vi "CUDA Toolkit Not Complex Graph.vi"(7 "nb_loop":i32=5, 8 "error in (no error)":errorcluster, 10 "B":refnum<class "Tensor.lvclass">, 11 "A":refnum<class "Tensor.lvclass">) -> (0 "error out":errorcluster, 3 "sum":sgl)   [LabVIEW 2020]
uses:
  Cuda/Source/Tensor.lvclass
  Cuda/Source/Methods/Functions/Numeric/SGL/Add Array Scalar(SGL).vi
  Cuda/Source/Methods/Functions/Numeric/SGL/Multiply Array Array(SGL).vi
  Cuda/Source/Methods/Functions/Numeric/SGL/Divide Array Array(SGL).vi
  Cuda/Source/Methods/Functions/Numeric/SGL/Add Array Element(SGL).vi
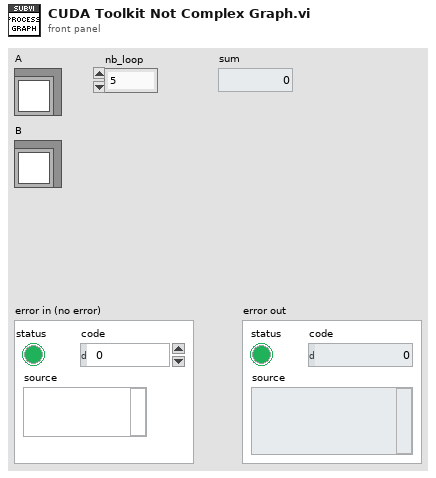
[diagram p1: front panel]
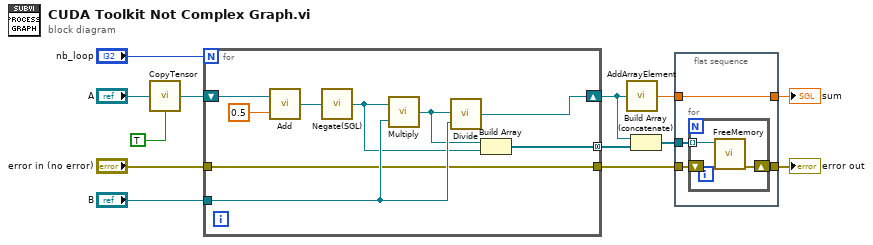
[diagram p0: block diagram]
diagram:
  n1 = call "CopyTensor.vi"("Tensor Src"="A", "copy data ?"=TRUE) -> ("Tensor Dst"=w9:refnum<class "Tensor.lvclass">)  [unwired: 13 in]
  n2 = for {
    N: "nb_loop" -> [_]
    tunnel: "B" -> [w20]
    shift-right: [w19] -> w5
    shift-left: w9 -> [w21]
    tunnel: "error in (no error)" -> [w17]
    tunnel: [w17] -> w7
    tunnel: [w14] -> w4 mode=concatenating
    n3 = call-poly "Add.vi"("y"=sgl 0.5, "x"=w21) -> ("x + y"=w18:refnum<class "Tensor.lvclass">)
    n4 = call "Negate(SGL).vi"("x"=w18) -> ("-x"=w15:refnum<class "Tensor.lvclass">)
    n5 = call-poly "Multiply.vi"("y"=w20, "x"=w15) -> ("x * y"=w16:refnum<class "Tensor.lvclass">)
    n6 = call-poly "Divide.vi"("y"=w20, "x"=w16) -> ("x / y"=w19:refnum<class "Tensor.lvclass">)
    n7 = Build Array(w16, w15) -> (w14:refnum<class "Tensor.lvclass">[])
  }
  n8 = call-poly "AddArrayElement.vi"("x"=w5) -> ("sum"=w1:sgl)
  n9 = Build Array (concatenate)(w5, w4) -> (w3:refnum<class "Tensor.lvclass">[])
  n10 = flat-sequence {
    tunnel: w7 -> [w26]
    tunnel: [w25] -> w6
    tunnel: w3 -> [w24]
    tunnel: [w23] -> w2
    tunnel: w1 -> [w23]
    frame #0 {
      n11 = for {
        shift-right: [w28] -> w25
        shift-left: w26 -> [w29]
        tunnel: w24 -> [w27] mode=indexing
        n12 = call "FreeMemory.vi"("error in"=w29, "Tensor in"=w27) -> ("error out"=w28:errorcluster)  [unwired: 9 in]
      }
    }
  }
  "error out" <- w6
  "sum" <- w2
